vi "GetParam.vi"(8 "error in (no error)":errorcluster caption="entrée d'erreur (pas d'erreur)", 11 "PredefinedSplit.lvclass":refnum<class "PredefinedSplit.lvclass">) -> (0 "error out":errorcluster caption="sortie d'erreur", 2 "PredefinedSplit":cluster{"test_fold":dbl[]}, 3 "PredefinedSplit.lvclass":refnum<class "PredefinedSplit.lvclass">)   [LabVIEW 2020, in "PredefinedSplit.lvclass"]
doc: "Get Parameters"
uses:
  PredefinedSplit.lvclass
  PredefinedSplit.lvclass/PredefinedSplit.ctl
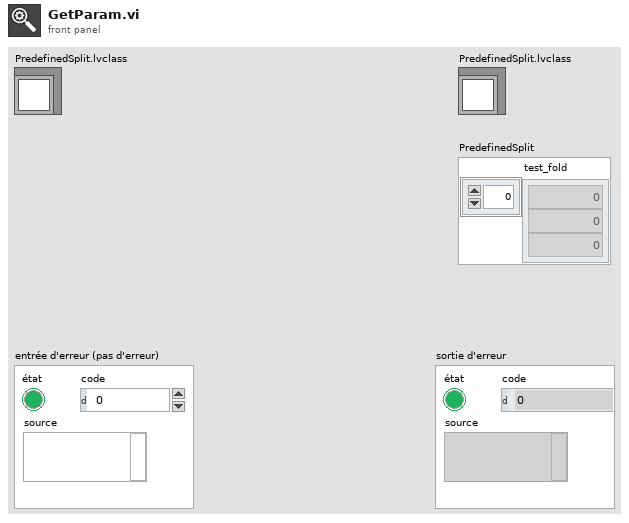
[diagram p1: front panel]
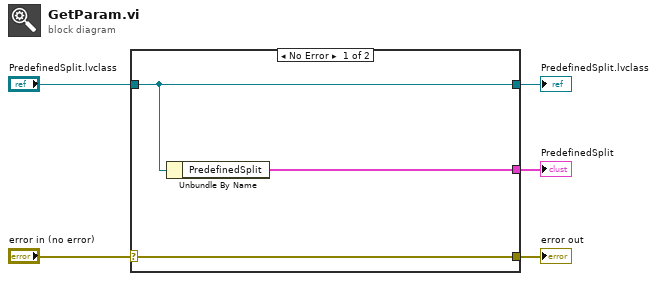
[diagram p0: block diagram]
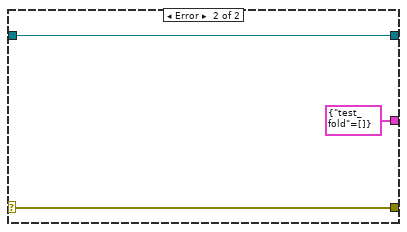
[diagram p2: hidden frame]
diagram:
  n1 = case shown="No Error" "error in (no error)" {
    selector: "error in (no error)" -> [w8 w10]
    tunnel: [w8 w10] -> w4
    tunnel: [w7 w11] -> w2
    tunnel: "PredefinedSplit.lvclass" -> [w7 w11]
    tunnel: [w6 cluster{"test_fold":dbl[]} {"test_fold"=[]} ("PredefinedSplit")] -> w1
    frame No Error {
      n2 = Unbundle By Name(w7) -> ("PredefinedSplit"=w6:cluster{"test_fold":dbl[]})
    }
    frame Error {
    }
  }
  "error out" <- w4
  "PredefinedSplit.lvclass" <- w2
  "PredefinedSplit" <- w1
